vi "Events.vi"(11 "ColumnPanel in":refnum<class "ColumnPanel.lvclass">) -> (2 "Events":T1)   [LabVIEW 2020, in "Conditum-Tools.lvlib" / "ColumnPanel.lvclass"]
uses:
  ColumnPanel.lvclass
  Events.ctl
  Field Event Data.ctl
  Field Config.ctl
  Conditum-Clone/Columns/Type/Type.lvclass
  Accessor Scope.ctl
  Property Update.ctl
  ColumnPanel.lvclass/ColumnPanel.ctl
  Conditum-Tools.lvlib
  Accessors.ctl
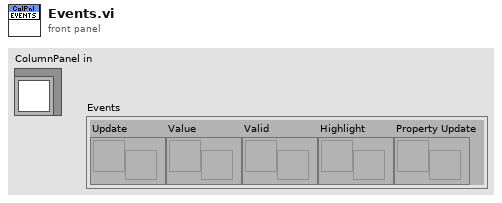
[diagram p1: front panel]
types:
  T1 = typedef "Conditum-Tools.lvlib/ColumnPanel.lvclass/Events.ctl" = cluster{"Update":refnum<user-event>, "Value":refnum<user-event>, "Valid":refnum<user-event>, "Highlight":refnum<user-event>, "Property Update":refnum<user-event>}
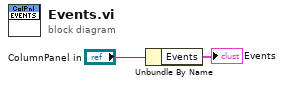
[diagram p0: block diagram]
diagram:
  n1 = Unbundle By Name("ColumnPanel in") -> ("Events"=→"Events":T1)
